vi "Read Array Key.vi"() -> (2 "def":dbl[](array[numeric]), 3 "abc":string[](array[string]))   [LabVIEW 2017]
uses:
  INI-Static-Variable-Support/LabVIEW-Config/Read Key (String).vi
  INI-Static-Variable-Support/LabVIEW-Config/Read Key (DBL).vi
  INI-Static-Variable-Support/LabVIEW-Config/Read Array Key (String).vi
  INI-Static-Variable-Support/LabVIEW-Config/Read Array Key (DBL).vi
  INI-Static-Variable-Support/LabVIEW-Config/LabVIEW-Config.lvlib
panel:
  out "Content":string[](array[string])
  out "def":dbl
  out "abc":string
  out "Key Names":string[](array[string])
  out "Section Names":string[](array[string])
  out "error out":errorcluster
  in  "error in (no error)":errorcluster
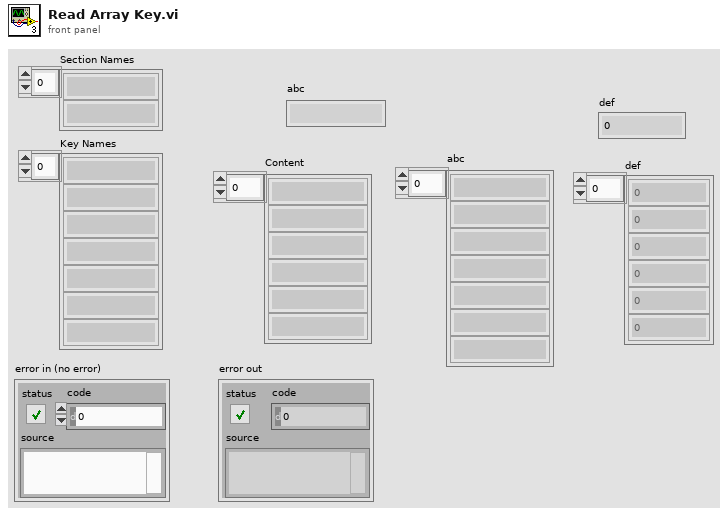
[diagram p1: front panel]
types:
  T1 = typedef "LabVIEW-Config.lvlib/Config.ctl" = cluster{"Path":path, "Lines":string[], "Tokens":enum8{"comment", "section", "key"}[], "Modified?":bool}
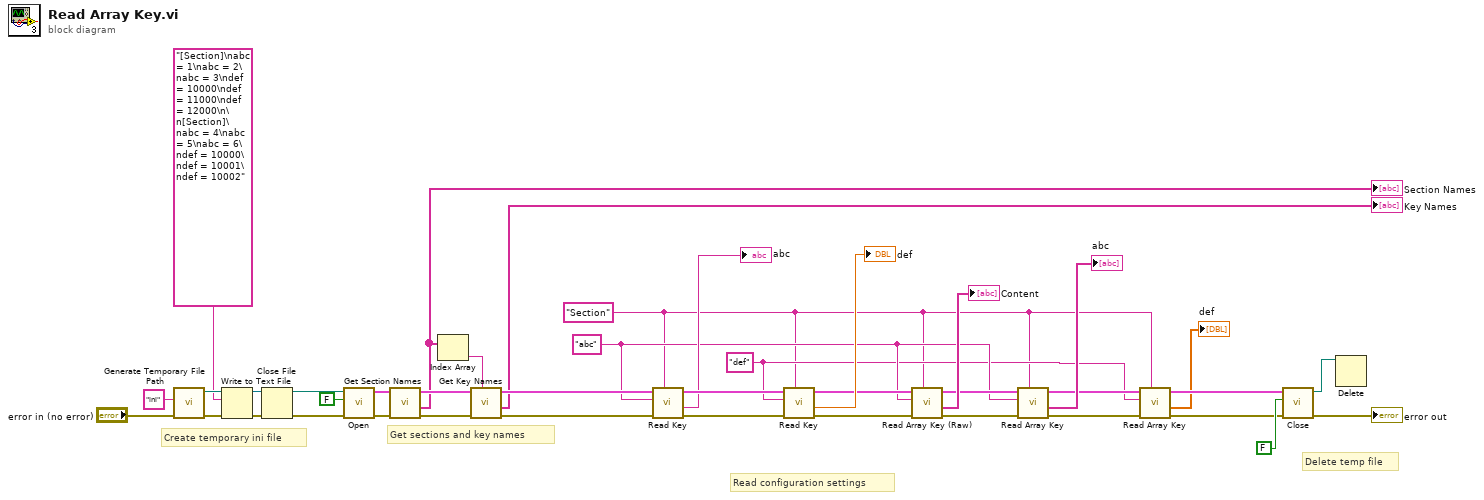
[diagram p0: block diagram]
diagram:
  w1 = "Section" ("Section Name")
  w3 = "def" ("Key Name")
  w9 = "abc" ("Key Name")
  # "Get sections and key names"
  # "Delete temp file"
  # "Read configuration settings"
  # "Create temporary ini file"
  n1 = call <vilib>:"Generate Temporary File Path.vi"("error in (no error)"="error in (no error)", "Temporary File Extension (tmp)"="ini") -> ("error out"=w34:errorcluster, "Unique Temporary File Path"=w31:path)  [unwired: 8 in]
  n2 = Write to Text File(file (use dialog)=w31, text="[Section]\nabc = 1\nabc = 2\nabc = 3\ndef = 10000\ndef = 11000\ndef = 12000\n\n[Section]\nabc = 4\nabc = 5\nabc = 6\ndef = 10000\ndef = 10001\ndef = 10002", error in=w34) -> (refnum out=w30:refnum<file>, error out=w32:errorcluster)  [unwired: 1 in, 1 out]
  n3 = Close File(refnum=w30, error in=w32) -> (path=w25:path, error out=w26:errorcluster)
  n4 = call "Open.vi"("error in (no error)"=w26, "Create if not exists? (T)"=FALSE, "Path"=w25) -> ("error out"=w38:errorcluster, "Config"=w23:T1)  [unwired: 5 in, 2 out]
  n5 = call "Get Section Names.vi"("error in (no error)"=w38, "Config in"=w23) -> ("error out"=w24:errorcluster, "Section Names"=w18:string[], "Config out"=w21:T1)  [unwired: 7 in]
  "Section Names" <- w18
  n6 = Index Array(array=w18) -> (element=w17:string)  [unwired: 1 in]
  n7 = call "Get Key Names.vi"("Section Name"=w17, "error in (no error)"=w24, "Config in"=w21) -> ("error out"=w22:errorcluster, "Key Names"=→"Key Names":string[], "Config out"=w20:T1)  [unwired: 5 in, 1 out]
  n8 = call-poly "Read Key.vi"("Section Name"=w1, "error in (no error)"=w22, "Key Name"=w9, "Config in"=w20) -> ("error out"=w37:errorcluster, "Value"=→"abc":string, "Config out"=w36:T1)  [unwired: 4 in, 1 out]
  n9 = call-poly "Read Key.vi"("Section Name"=w1, "error in (no error)"=w37, "Key Name"=w3, "Config in"=w36) -> ("error out"=w13:errorcluster, "Value"=→"def":dbl, "Config out"=w14:T1)  [unwired: 4 in, 1 out]
  n10 = call "Read Array Key (Raw).vi"("Section Name"=w1, "error in (no error)"=w13, "Key Name"=w9, "Config in"=w14) -> ("error out"=w12:errorcluster, "Content"=→"Content":string[], "Config out"=w10:T1)  [unwired: 4 in, 1 out]
  n11 = call-poly "Read Array Key.vi"("Section Name"=w1, "error in (no error)"=w12, "Key Name"=w9, "Config in"=w10) -> ("error out"=w7:errorcluster, "Value"=→"abc":string[], "Config out"=w6:T1)  [unwired: 4 in, 1 out]
  n12 = call-poly "Read Array Key.vi"("Section Name"=w1, "error in (no error)"=w7, "Key Name"=w3, "Config in"=w6) -> ("error out"=w4:errorcluster, "Value"=→"def":dbl[], "Config out"=w5:T1)  [unwired: 4 in, 1 out]
  n13 = call "Close.vi"("error in (no error)"=w4, "Write if modified? (T)"=FALSE, "Config"=w5) -> ("error out"=→"error out":errorcluster, "Path"=w28:path)  [unwired: 7 in]
  n14 = Delete(path (use dialog)=w28) -> ()  [unwired: 4 in, 3 out]
